vi "visitor4.vi"() -> ()   [LabVIEW 2014]
uses:
  <vilib>/express/express arith-compare/Formula/XNode/ExpressFormulaBlockNode.xnode
  <vilib>/ptbypt/NI_PtbyPt.lvlib
panel:
  in  "Simulation Speed":i8(knob) min=0 max=8 step=1 scale=0.0..8.0
  in  "Dial 4":i8(knob)=1 min=1 max=2 step=1 scale=0.0..3.0
  in  "Dial 3":i8(knob)=1 min=1 max=2 step=1 scale=0.0..3.0
  in  "Dial 2":i8(knob)=1 min=1 max=2 step=1 scale=0.0..3.0
  in  "Dial":i8(knob)=1 min=1 max=2 step=1 scale=0.0..3.0
  out "HIGH POOL TOP RAD":bool
  out "Pool Top Radiation (µSv/h)":dbl
  out "RG":dbl format="%0_5g"
  out "SH":dbl format="%0_5g"
  out "SF":dbl format="%0_5g"
  out "TR":dbl format="%0_5g"
  in  "ACK":bool
  out "Control Rod Speed (mm/s)":dbl
  out "lograte (%/s)":dbl
  out "Reactor Period (s)":dbl
  in  "SCRAM RESET":bool
  out "Reactor Period":dbl(slide) scale=0.0..100.0
  out "over power":bool
  out "high water temp":bool
  out "high fuel temp":bool
  out "short period":bool
  out "manual SCRAM":bool
  in  "MANUAL SYSTEM TRIP":bool
  in  "Test Short Period":dbl(knob) scale=0.0..100.0
  in  "Test Water Temp":dbl(knob) scale=0.0..100.0
  in  "Test Fuel Temp":dbl(knob) scale=0.0..600.0
  in  "Test Reactor Power":dbl(knob) scale=0.0..125.0
  out "Average Rod Reactivity ($)":dbl
  out "RG ($)":dbl
  out "SH ($)":dbl
  out "SF ($)":dbl
  out "TR ($)":dbl format="%_6g"
  out "Reactor Simulation Chart":T1(graph)
  out "Reactor Power (%)":dbl
  out "Water Temp":dbl
  out "Fuel Temp":dbl
  out "Reactor Power (w)":dbl
  out "Average Control Rod Position (mm)":dbl
  in  "Down Button 4":bool
  in  "Down Button 3":bool
  in  "Down Button 2":bool
  in  "Down Button":bool
  in  "Up Button 3":bool
  in  "Up Button 2":bool
  in  "Up Button":bool
  in  "Up Button":bool
  in  "stop":bool
  out "Tank 12":dbl(slide) scale=0.0..400.0
  out "Tank 11":dbl(slide) scale=0.0..400.0
  out "Tank 10":dbl(slide) scale=0.0..400.0
  out "Tank 9":dbl(slide) scale=0.0..400.0
  out "Tank 8":dbl(slide) scale=0.0..400.0
  out "Tank 7":dbl(slide) scale=0.0..400.0
  out "Tank 6":dbl(slide) scale=0.0..400.0
  out "Tank 5":dbl(slide) scale=0.0..400.0
  out "Tank 4":dbl(slide) scale=0.0..400.0
  out "Tank 3":dbl(slide) scale=0.0..400.0
  out "Tank 2":dbl(slide) scale=0.0..400.0
  out "Tank":dbl(slide) scale=0.0..400.0
  # "Real Time"
  # "Slow"
  # "Fast"
  # "0.5s"
  # "2s"
  # "0.1s"
  # "3s"
  # "4s"
  # "0.05s"
  # "5s"
  # "0.01s"
  # "3-"
  # "4-"
  # "FIELD"
  # "TEST"
  # "FIELD"
  # "TEST"
  # "FIELD"
  # "TEST"
  # "FIELD"
  # "TEST"
  # "5-"
  # "6-"
  # "7-"
  # "8-"
  # "10-"
  # "15-"
  # "20-"
  # "30-"
  # "50-"
  # "100-"
  # "INF-"
  # "-100-"
  # "Rod SF"
  # "Rod SH"
  # "Rod RG"
  # "-50-"
  # "Rod TR"
  # "-30-"
  # "0"
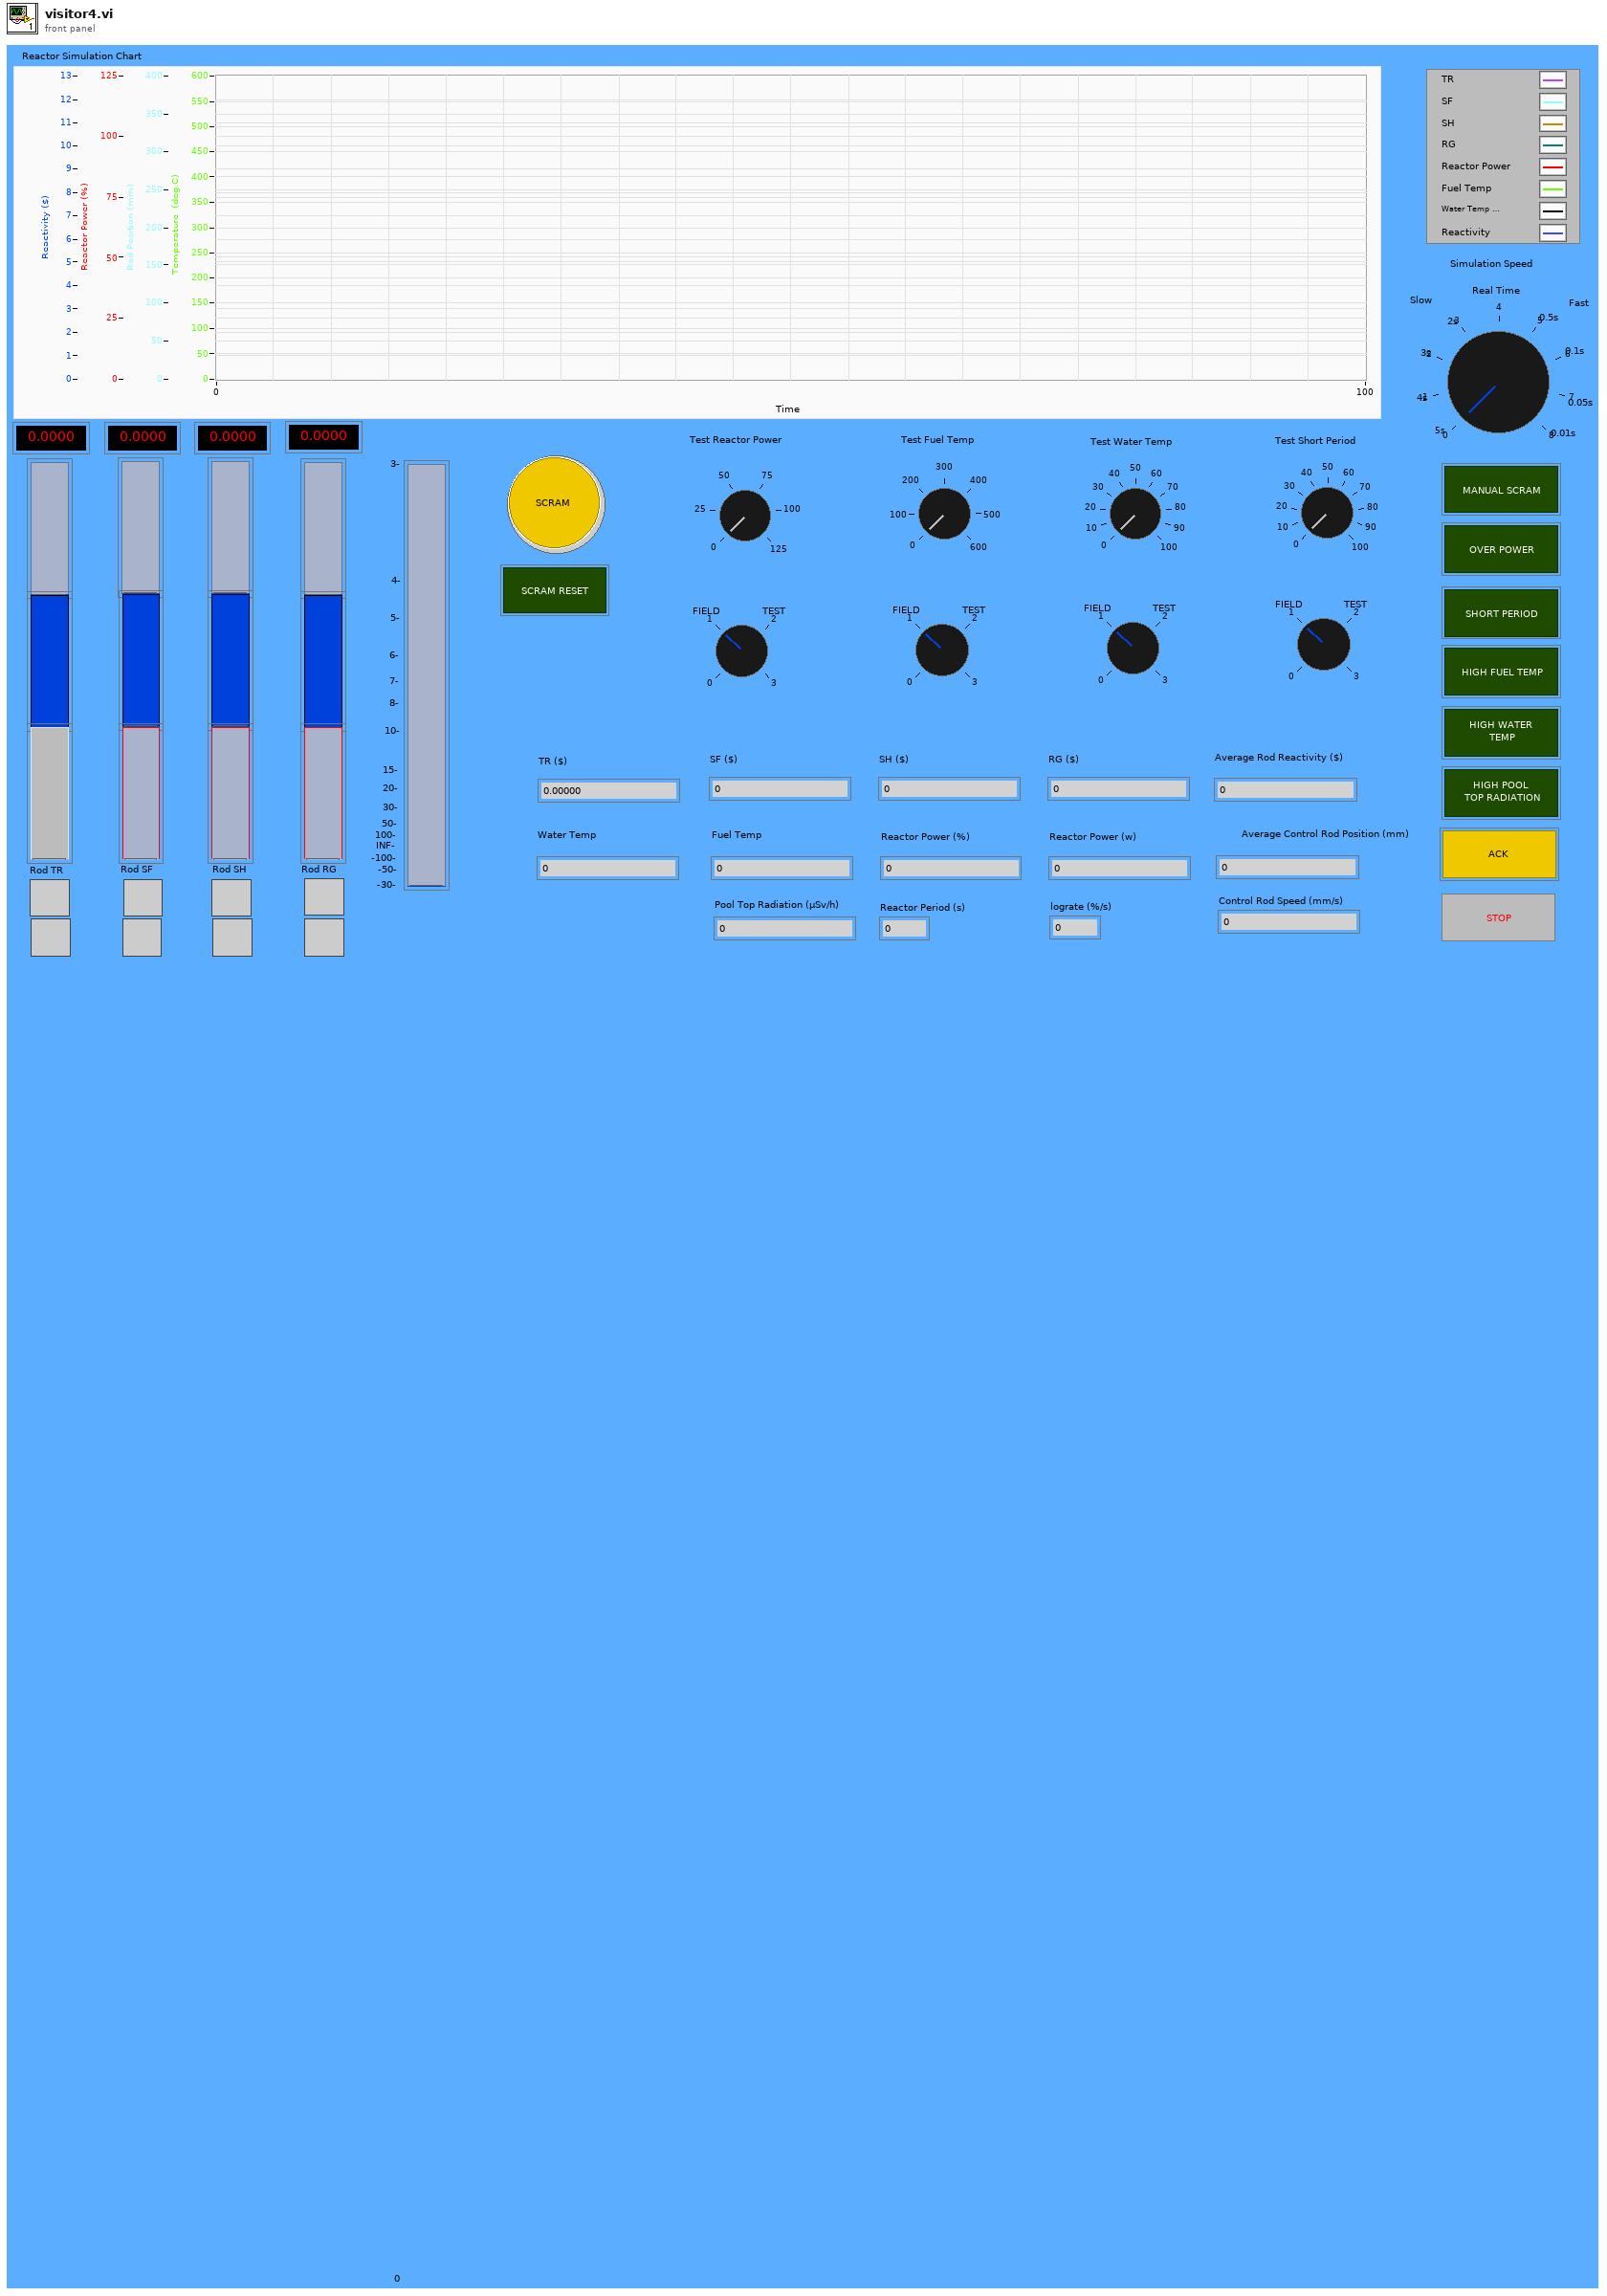
[diagram p1: front panel]
types:
  T1 = cluster{"TR (mm)":dbl, "SF (mm)":dbl, "SH (mm)":dbl, "RG (mm)":dbl, dbl, "Result":dbl, "Result":dbl, dbl}
  T2 = cluster{"upper limit":dbl, "upper limit":dbl, "upper limit":dbl, "upper limit":dbl, "Test Reactor Power":dbl, "Test Fuel Temp":dbl, "Test Water Temp":dbl, "upper limit":dbl}
  T3 = typedef "Sound Output Task ID.ctl" = u32
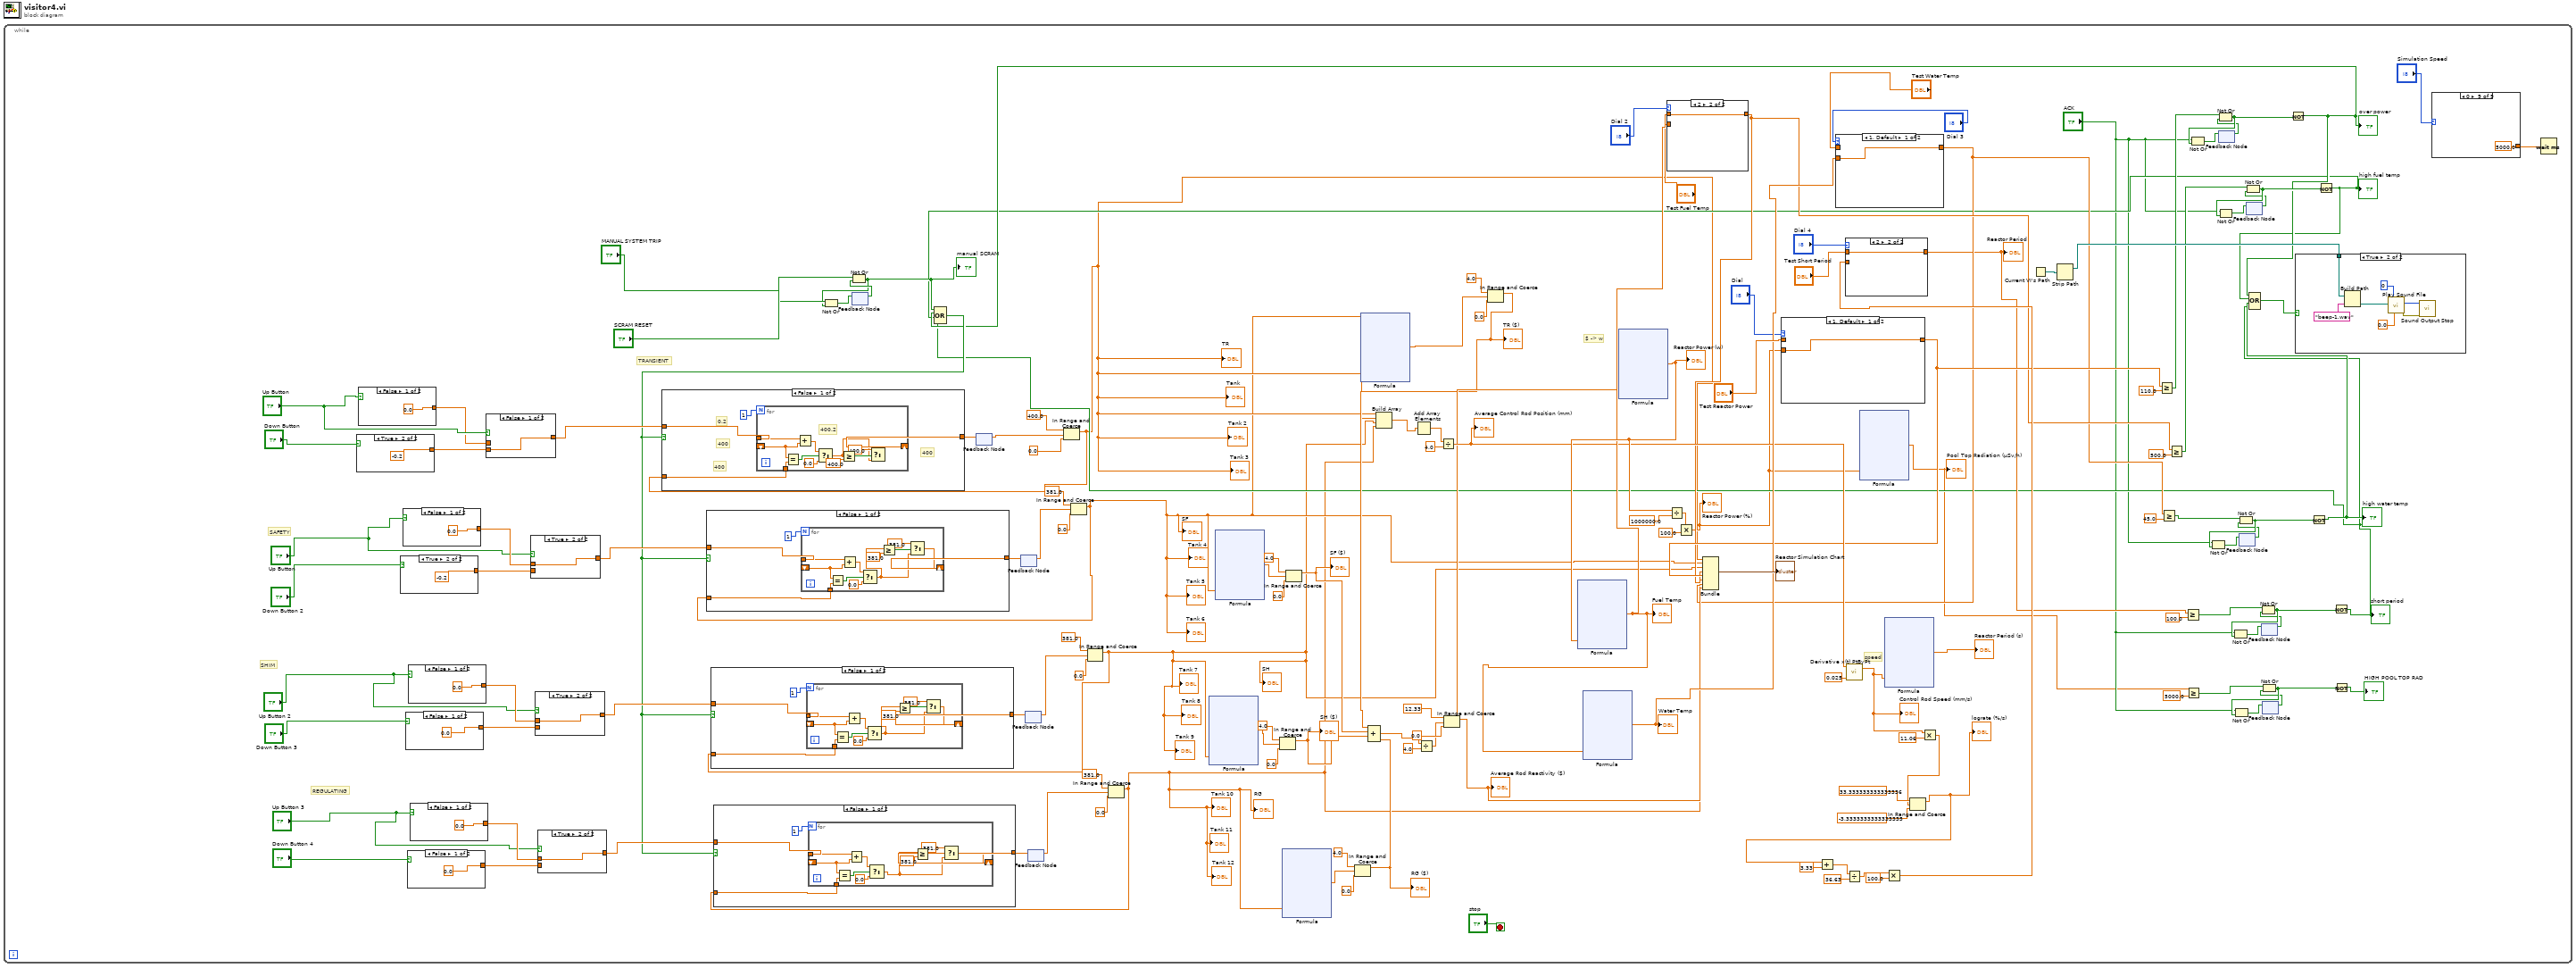
[diagram p0: block diagram]
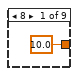
[diagram p2: hidden frame]
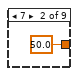
[diagram p3: hidden frame]
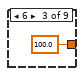
[diagram p4: hidden frame]
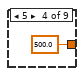
[diagram p5: hidden frame]
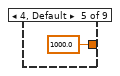
[diagram p6: hidden frame]
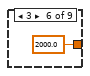
[diagram p7: hidden frame]
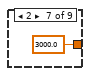
[diagram p8: hidden frame]
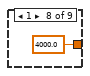
[diagram p9: hidden frame]
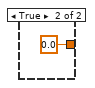
[diagram p10: hidden frame]
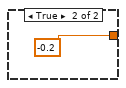
[diagram p12: hidden frame]
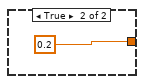
[diagram p13: hidden frame]
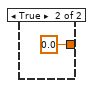
[diagram p14: hidden frame]
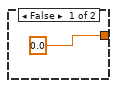
[diagram p16: hidden frame]
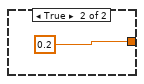
[diagram p17: hidden frame]
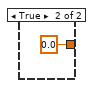
[diagram p18: hidden frame]
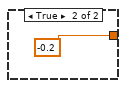
[diagram p20: hidden frame]
diagram:
  n1 = while {
    stop <- "stop" stop-if-true
    # "speed"
    # "$ -> w"
    # "REGULATING"
    # "SHIM"
    # "SAFETY"
    # "TRANSIENT"
    n2 = case shown="True" "Down Button" {
      tunnel: [0.0 -0.2] -> w141
      frame False {
      }
      frame True {
      }
    }
    n3 = case shown="False" "Up Button" {
      tunnel: [0.0 0.2] -> w49
      frame False {
      }
      frame True {
      }
    }
    n4 = case shown="True" "Down Button 2" {
      tunnel: [0.0 -0.2] -> w40
      frame False {
      }
      frame True {
      }
    }
    n5 = case shown="False" "Up Button" {
      tunnel: [0.0 0.2] -> w39
      frame False {
      }
      frame True {
      }
    }
    n6 = case shown="False" "Down Button 3" {
      tunnel: [0.0 -0.2] -> w46
      frame False {
      }
      frame True {
      }
    }
    n7 = case shown="False" "Down Button 4" {
      tunnel: [0.0 -0.2] -> w34
      frame False {
      }
      frame True {
      }
    }
    n8 = case shown="False" "Up Button 2" {
      tunnel: [0.0 0.2] -> w45
      frame False {
      }
      frame True {
      }
    }
    n9 = case shown="False" "Up Button 3" {
      tunnel: [0.0 0.2] -> w33
      frame False {
      }
      frame True {
      }
    }
    n10 = case shown="False" "Up Button" {
      tunnel: [w323 w324] -> w48
      tunnel: w49 -> [_ w324]
      tunnel: w141 -> [w323 _]
      frame False {
      }
      frame True {
      }
    }
    n11 = case shown="True" "Up Button" {
      tunnel: [w200 w201] -> w38
      tunnel: w39 -> [_ w201]
      tunnel: w40 -> [w200 _]
      frame False {
      }
      frame True {
      }
    }
    n12 = case shown="True" "Up Button 2" {
      tunnel: [w222 w223] -> w44
      tunnel: w45 -> [_ w223]
      tunnel: w46 -> [w222 _]
      frame False {
      }
      frame True {
      }
    }
    n13 = case shown="True" "Up Button 3" {
      tunnel: [w178 w179] -> w32
      tunnel: w33 -> [_ w179]
      tunnel: w34 -> [w178 _]
      frame False {
      }
      frame True {
      }
    }
    n14 = feedback #1() -> (w69:bool)  [unwired: 1 in]
    n15 = Not Or(1:w69, 2:"SCRAM RESET") -> (0:w28:bool)
    "manual SCRAM" <- w28
    n16 = Not Or ("Not Or 2")(1:w28, 2:"MANUAL SYSTEM TRIP") -> (0:w68:bool)
    n17 = feedback-in #1 ("12")(w68) -> ()
    n18 = feedback #2() -> (w8:dbl)  [unwired: 1 in]
    n19 = feedback #3() -> (w1:dbl)  [unwired: 1 in]
    n20 = feedback #4() -> (w5:dbl)  [unwired: 1 in]
    n21 = feedback #5() -> (w3:dbl)  [unwired: 1 in]
    n22 = In Range and Coerce(upper limit=400.0, x=w8, lower limit=0.0) -> (coerced(x)=w7:dbl)  [unwired: 1 out]
    "Tank" <- w7
    "Tank 2" <- w7
    "Tank 3" <- w7
    "TR" <- w7
    n23 = In Range and Coerce(upper limit=381.0, x=w1, lower limit=0.0) -> (coerced(x)=w6:dbl)  [unwired: 1 out]
    "Tank 4" <- w6
    "Tank 5" <- w6
    "Tank 6" <- w6
    "SF" <- w6
    n24 = In Range and Coerce(upper limit=381.0, x=w5, lower limit=0.0) -> (coerced(x)=w4:dbl)  [unwired: 1 out]
    "Tank 7" <- w4
    "Tank 8" <- w4
    "Tank 9" <- w4
    "SH" <- w4
    n25 = In Range and Coerce(upper limit=381.0, x=w3, lower limit=0.0) -> (coerced(x)=w2:dbl)  [unwired: 1 out]
    "Tank 10" <- w2
    "Tank 11" <- w2
    "Tank 12" <- w2
    "RG" <- w2
    n26 = xnode "Formula"("X1"=w4) -> ("Result"=w50:dbl)  [unwired: 1 in, 1 out]
    n27 = xnode "Formula"("X1"=w6) -> ("Result"=w55:dbl)  [unwired: 1 in, 1 out]
    n28 = In Range and Coerce(upper limit=4.0, x=w50, lower limit=0.0) -> (coerced(x)=w51:dbl)  [unwired: 1 out]
    "SH ($)" <- w51
    n29 = xnode "Formula"("X1"=w2) -> ("Result"=w58:dbl)  [unwired: 1 in, 1 out]
    n30 = In Range and Coerce(upper limit=4.0, x=w55, lower limit=0.0) -> (coerced(x)=w54:dbl)  [unwired: 1 out]
    "SF ($)" <- w54
    n31 = In Range and Coerce(upper limit=4.0, x=w58, lower limit=0.0) -> (coerced(x)=w59:dbl)  [unwired: 1 out]
    "RG ($)" <- w59
    n32 = xnode "Formula"("X1"=w7) -> ("Result"=w63:dbl)  [unwired: 1 in, 1 out]
    n33 = Build Array(w7, w6, w4, w2) -> (w132:dbl[])
    n34 = Add Array Elements(numeric array=w132) -> (sum=w131:dbl)
    n35 = Divide(x=w131, y=4.0) -> (x/y=w115:dbl)
    "Average Control Rod Position (mm)" <- w115
    n36 = In Range and Coerce(upper limit=4.0, x=w63, lower limit=0.0) -> (coerced(x)=w62:dbl)  [unwired: 1 out]
    "TR ($)" <- w62
    n37 = Compound Arithmetic op=ADD(w62, w54, w51, w59) -> (w124:dbl)
    n38 = Divide(x=w124, y=4.0) -> (x/y=w105:dbl)
    n39 = In Range and Coerce(upper limit=12.33, x=w105, lower limit=0.0) -> (coerced(x)=w106:dbl)  [unwired: 1 out]
    "Average Rod Reactivity ($)" <- w106
    n40 = xnode "Formula"("X1"=w106) -> ("Result"=w123:dbl)  [unwired: 1 in, 1 out]
    "Reactor Power (w)" <- w123
    n41 = xnode "Formula"("X1"=w123) -> ("Result"=w121:dbl)  [unwired: 1 in, 1 out]
    "Fuel Temp" <- w121
    n42 = xnode "Formula"("X1"=w121) -> ("Result"=w118:dbl)  [unwired: 1 in, 1 out]
    "Water Temp" <- w118
    n43 = case shown="2" "Dial 2" {
      tunnel: "Test Fuel Temp" -> [_ w256]
      tunnel: [w255 w256] -> w89
      tunnel: w121 -> [w255 _]
      frame 1, Default {
      }
      frame 2 {
      }
    }
    n44 = Divide(x=w123, y=1000000.0) -> (x/y=w129:dbl)
    n45 = Multiply(x=w129, y=100.0) -> (x*y=w23:dbl)
    "Reactor Power (%)" <- w23
    n46 = case shown="1, Default" "Dial" {
      tunnel: "Test Reactor Power" -> [_ w258]
      tunnel: [w257 w258] -> w96
      tunnel: w23 -> [w257 _]
      frame 1, Default {
      }
      frame 2 {
      }
    }
    n47 = case shown="1, Default" "Dial 3" {
      tunnel: "Test Water Temp" -> [_ w254]
      tunnel: [w253 w254] -> w78
      tunnel: w118 -> [w253 _]
      frame 1, Default {
      }
      frame 2 {
      }
    }
    n48 = Bundle("upper limit"=w7, "upper limit"=w6, "upper limit"=w4, "upper limit"=w2, "Test Reactor Power"=w96, "Test Fuel Temp"=w89, "Test Water Temp"=w78, "upper limit"=w106) -> (→"Reactor Simulation Chart":T2)  [unwired: 1 in]
    n49 = call <vilib>:"Derivative x(t) PtByPt.vi"("dt"=0.025, "x"=w115) -> ("dx/dt"=w104:dbl)  [unwired: 2 in, 1 out]
    "Control Rod Speed (mm/s)" <- w104
    n50 = xnode "Formula"("X1"=w23) -> ("Result"=w15:dbl)  [unwired: 1 in, 1 out]
    "Pool Top Radiation (µSv/h)" <- w15
    n51 = xnode "Formula"("X1"=w104) -> ("Result"=→"Reactor Period (s)":dbl)  [unwired: 1 in, 1 out]
    n52 = Multiply(x=w104, y=11.06) -> (x*y=w99:dbl)
    n53 = In Range and Coerce(upper limit=33.333333333333336, x=w99, lower limit=-3.3333333333333335) -> (coerced(x)=w98:dbl)  [unwired: 1 out]
    "lograte (%/s)" <- w98
    n54 = Add(x=w98, y=3.33) -> (x+y=w111:dbl)
    n55 = Divide(x=w111, y=36.63) -> (x/y=w103:dbl)
    n56 = Multiply(x=w103, y=100.0) -> (x*y=w100:dbl)
    n57 = case shown="2" "Dial 4" {
      tunnel: "Test Short Period" -> [_ w252]
      tunnel: [w251 w252] -> w70
      tunnel: w100 -> [w251 _]
      frame 1, Default {
      }
      frame 2 {
      }
    }
    "Reactor Period" <- w70
    n58 = Current VI's Path() -> (path=w91:path)
    n59 = Strip Path(path=w91) -> (stripped path=w92:path)  [unwired: 1 out]
    n60 = Greater Or Equal?(x=w96, y=110.0) -> (x >= y?=w88:bool)
    n61 = Greater Or Equal?(x=w78, y=45.0) -> (x >= y?=w76:bool)
    n62 = Greater Or Equal?(x=w89, y=500.0) -> (x >= y?=w84:bool)
    n63 = Greater Or Equal?(x=w70, y=100.0) -> (x >= y?=w71:bool)
    n64 = Greater Or Equal?(x=w15, y=5000.0) -> (x >= y?=w18:bool)
    n65 = feedback #6 ("Feedback Node 7")() -> (w94:bool)  [unwired: 1 in]
    n66 = Not Or ("Not Or 13")(1:w94, 2:w88) -> (0:w95:bool)
    n67 = Not Or ("Not Or 14")(1:w95, 2:"ACK") -> (0:w93:bool)
    n68 = feedback-in #6 ("18")(w93) -> ()
    n69 = feedback #7 ("Feedback Node 7")() -> (w81:bool)  [unwired: 1 in]
    n70 = Not Or ("Not Or 13")(1:w81, 2:w76) -> (0:w82:bool)
    n71 = Not Or ("Not Or 14")(1:w82, 2:"ACK") -> (0:w80:bool)
    n72 = feedback-in #7 ("18")(w80) -> ()
    n73 = feedback #8 ("Feedback Node 7")() -> (w86:bool)  [unwired: 1 in]
    n74 = Not Or ("Not Or 13")(1:w86, 2:w84) -> (0:w87:bool)
    n75 = Not Or ("Not Or 14")(1:w87, 2:"ACK") -> (0:w85:bool)
    n76 = feedback-in #8 ("18")(w85) -> ()
    n77 = feedback #9 ("Feedback Node 7")() -> (w73:bool)  [unwired: 1 in]
    n78 = Not Or ("Not Or 13")(1:w73, 2:w71) -> (0:w74:bool)
    n79 = Not Or ("Not Or 14")(1:w74, 2:"ACK") -> (0:w72:bool)
    n80 = feedback-in #9 ("18")(w72) -> ()
    n81 = feedback #10 ("Feedback Node 7")() -> (w20:bool)  [unwired: 1 in]
    n82 = Not Or ("Not Or 13")(1:w20, 2:w18) -> (0:w21:bool)
    n83 = Not Or ("Not Or 14")(1:w21, 2:"ACK") -> (0:w19:bool)
    n84 = feedback-in #10 ("18")(w19) -> ()
    n85 = Not ("Not 6")(x=w95) -> (.not. x?=w26:bool)
    "over power" <- w26
    n86 = Not ("Not 6")(x=w82) -> (.not. x?=w77:bool)
    "high water temp" <- w77
    n87 = Not ("Not 6")(x=w87) -> (.not. x?=w25:bool)
    "high fuel temp" <- w25
    n88 = Not ("Not 6")(x=w74) -> (.not. x?=w24:bool)
    "short period" <- w24
    n89 = Compound Arithmetic op=OR(w28, w26, w25, w24) -> (w27:bool)
    n90 = case shown="False" w27 {
      tunnel: w48 -> [w231 _]
      tunnel: [w229 0.0] -> w47
      tunnel: w7 -> [w228 _]
      frame False {
        # "0.2"
        # "400"
        # "400"
        # "400"
        n91 = for {
          N: 1 -> [_]
          tunnel: w231 -> [w242]
          shift-right: [w236] -> w229
          shift-left: _ -> [w238]
          tunnel: w228 -> [w237]
          # "400.2"
          n92 = Equal?(x=w238, y=w237) -> (x = y?=w239:bool)
          n93 = Add(x=w242, y=w238) -> (x+y=w241:dbl)
          n94 = Select(t=w241, s=w239, f=0.0) -> (s? t:f=w232:dbl)
          n95 = Greater Or Equal?(x=w232, y=400.0) -> (x >= y?=w234:bool)
          n96 = Select(t=400.0, s=w234, f=w232) -> (s? t:f=w236:dbl)
        }
      }
      frame True {
      }
    }
    n97 = case shown="False" w27 {
      tunnel: w38 -> [w187 _]
      tunnel: [w185 0.0] -> w37
      tunnel: w6 -> [w184 _]
      frame False {
        n98 = for {
          N: 1 -> [_]
          tunnel: w187 -> [w198]
          shift-right: [w189] -> w185
          shift-left: _ -> [w194]
          tunnel: w184 -> [w193]
          n99 = Equal?(x=w194, y=w193) -> (x = y?=w195:bool)
          n100 = Add(x=w198, y=w194) -> (x+y=w197:dbl)
          n101 = Select(t=w197, s=w195, f=0.0) -> (s? t:f=w188:dbl)
          n102 = Greater Or Equal?(x=w188, y=381.0) -> (x >= y?=w191:bool)
          n103 = Select(t=381.0, s=w191, f=w188) -> (s? t:f=w189:dbl)
        }
      }
      frame True {
      }
    }
    n104 = case shown="False" w27 {
      tunnel: w44 -> [w209 _]
      tunnel: [w207 0.0] -> w43
      tunnel: w4 -> [w206 _]
      frame False {
        n105 = for {
          N: 1 -> [_]
          tunnel: w209 -> [w220]
          shift-right: [w212] -> w207
          shift-left: _ -> [w216]
          tunnel: w206 -> [w215]
          n106 = Equal?(x=w216, y=w215) -> (x = y?=w217:bool)
          n107 = Add(x=w220, y=w216) -> (x+y=w219:dbl)
          n108 = Select(t=w219, s=w217, f=0.0) -> (s? t:f=w210:dbl)
          n109 = Greater Or Equal?(x=w210, y=381.0) -> (x >= y?=w211:bool)
          n110 = Select(t=381.0, s=w211, f=w210) -> (s? t:f=w212:dbl)
        }
      }
      frame True {
      }
    }
    n111 = case shown="False" w27 {
      tunnel: w32 -> [w165 _]
      tunnel: [w163 0.0] -> w31
      tunnel: w2 -> [w162 _]
      frame False {
        n112 = for {
          N: 1 -> [_]
          tunnel: w165 -> [w176]
          shift-right: [w167] -> w163
          shift-left: _ -> [w172]
          tunnel: w162 -> [w171]
          n113 = Equal?(x=w172, y=w171) -> (x = y?=w173:bool)
          n114 = Add(x=w176, y=w172) -> (x+y=w175:dbl)
          n115 = Select(t=w175, s=w173, f=0.0) -> (s? t:f=w166:dbl)
          n116 = Greater Or Equal?(x=w166, y=381.0) -> (x >= y?=w169:bool)
          n117 = Select(t=381.0, s=w169, f=w166) -> (s? t:f=w167:dbl)
        }
      }
      frame True {
      }
    }
    n118 = feedback-in #2(w47) -> ()
    n119 = feedback-in #3(w37) -> ()
    n120 = feedback-in #4(w43) -> ()
    n121 = feedback-in #5(w31) -> ()
    n122 = Compound Arithmetic op=OR(w26, w25, w77, w24) -> (w83:bool)
    n123 = case "Case Structure 31" shown="True" w83 {
      tunnel: w92 -> [_ w246]
      frame False {
      }
      frame True {
        n124 = Build Path ("Build Path 2")(base path=w246, name or relative path="beep-1.wav") -> (appended path=w249:path)
        n125 = call <vilib>:"Play Sound File.vi"("timeout (sec)"=0.0, "path"=w249, "device ID"=u32 0) -> ("error out"=w244:errorcluster, "task ID"=w245:T3)  [unwired: 7 in]
        n126 = call <vilib>:"Sound Output Stop.vi"("error in (no error)"=w244, "task ID"=w245) -> ()  [unwired: 8 in, 2 out]
      }
    }
    n127 = Not ("Not 6")(x=w21) -> (.not. x?=→"HIGH POOL TOP RAD":bool)
    n128 = case shown="0" "Simulation Speed" {
      tunnel: [10.0 50.0 100.0 500.0 1000.0 2000.0 3000.0 4000.0 5000.0] -> w9
      frame 8 {
      }
      frame 7 {
      }
      frame 6 {
      }
      frame 5 {
      }
      frame 4, Default {
      }
      frame 3 {
      }
      frame 2 {
      }
      frame 1 {
      }
      frame 0 {
      }
    }
    n129 = Wait (ms)(milliseconds to wait=w9) -> ()  [unwired: 1 out]
  }
